vi "read field - fast.vi"(8 "error in (no error)":errorcluster, 11 "VISA resource name":refnum<visa-resource-name>="GPIB0::2::INSTR") -> (0 "error out":errorcluster, 2 "Current field (T)":dbl[unit], 3 "VISA resource name out":refnum<visa-resource-name>)   [LabVIEW 2012, in "Varian.lvlib"]
uses:
  Varian.lvlib
  Fluke Multimeter/Fluke 8840/Fluke 8840.lvlib
panel:
  out "unit":string
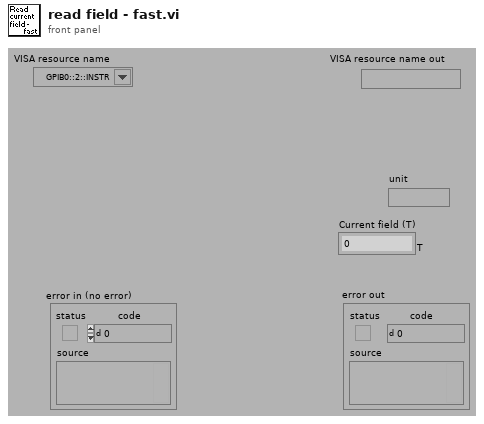
[diagram p1: front panel]
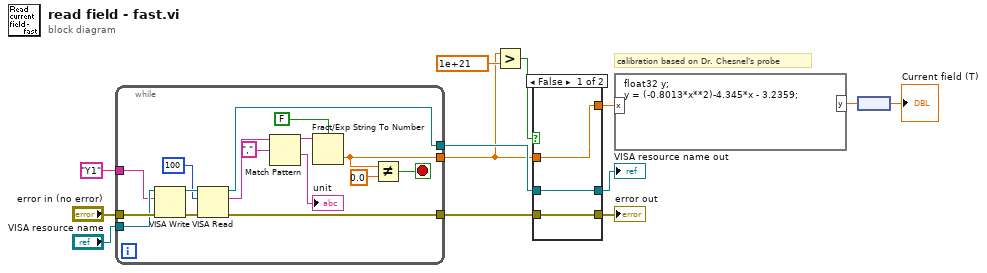
[diagram p0: block diagram]
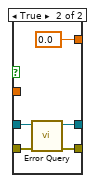
[diagram p2: hidden frame]
diagram:
  # "calibration based on Dr. Chesnel's probe"
  n1 = while {
    tunnel: "error in (no error)" -> [w29]
    tunnel: "VISA resource name" -> [w28]
    tunnel: [w20] -> w7
    tunnel: [w19] -> w6
    tunnel: [w14] -> w5
    tunnel: "Y1" -> [w17]
    stop <- w16 stop-if-true
    n2 = VISA Write(VISA resource name=w28, write buffer=w17, error in (no error)=w29) -> (VISA resource name out=w26:refnum<visa-resource-name>, error out=w27:errorcluster)  [unwired: 1 out]
    n3 = VISA Read(VISA resource name=w26, byte count=100, error in (no error)=w27) -> (VISA resource name out=w19:refnum<visa-resource-name>, read buffer=w21:string, error out=w20:errorcluster)  [unwired: 1 out]
    n4 = Match Pattern(string=w21, regular expression=",") -> (before substring=w23:string, after substring=→"unit":string)  [unwired: 3 out]
    n5 = Fract/Exp String To Number(use system decimal point (T)=FALSE, string=w23) -> (number=w14:dbl)  [unwired: 3 out]
    n6 = Not Equal?(x=w14, y=0.0) -> (x != y?=w16:bool)
  }
  n7 = Greater?(x=w5, y=1e+21) -> (0:w10:bool)
  n8 = case shown="False" w10 {
    tunnel: [w32 0.0] -> w2
    tunnel: [w31 w36] -> w9
    tunnel: [w30 w35] -> w8
    tunnel: w7 -> [w30 w34]
    tunnel: w6 -> [w31 w33]
    tunnel: w5 -> [w32 _]
    frame False {
    }
    frame True {
      n9 = call "Error Query.vi"("error in (no error)"=w34, "VISA resource name"=w33) -> ("error out"=w35:errorcluster, "VISA resource name out"=w36:refnum<visa-resource-name>)  [unwired: 1 in, 7 out]
    }
  }
  "error out" <- w8
  "VISA resource name out" <- w9
  n10 = formula code="float32 y;\ny = (-0.8013*x**2)-4.345*x - 3.2359;"("x"=w2) -> ("y"=w1:sgl)
  n11 = node(w1) -> (→"Current field (T)":sgl[unit])
